vi "Create Path URL.vi"(6 "Weight":i32=5, 7 "Path Collor":u32(colorbox)=16715776, 8 "Long Point 2":string, 9 "Lat Point 2":string, 10 "Long Point 1":string, 11 "Lat Point 1":string) -> (3 "String 4":string)   [LabVIEW 2012]
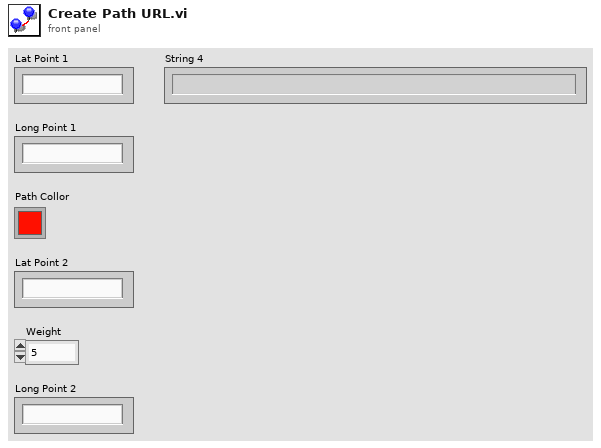
[diagram p1: front panel]
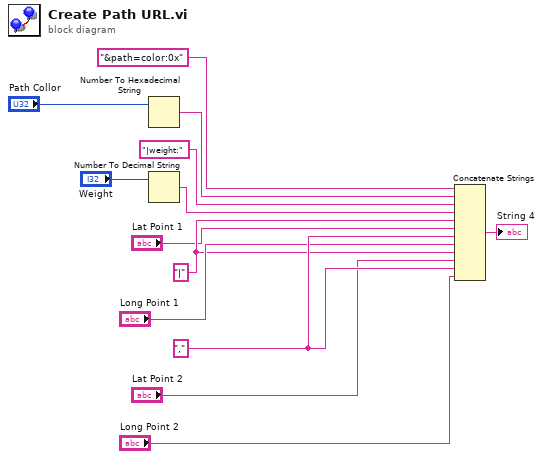
[diagram p0: block diagram]
diagram:
  w13 = "," ("string")
  w11 = "|"
  n1 = Number To Hexadecimal String(2:"Path Collor") -> (0:w3:string)  [unwired: 1 in]
  n2 = Number To Decimal String(number="Weight") -> (decimal integer string=w6:string)  [unwired: 1 in]
  n3 = Concatenate Strings("&path=color:0x" ("string"), w3, "|weight:", w6, w11, "Lat Point 1", w13, "Long Point 1", w11, "Lat Point 2", w13, "Long Point 2") -> (→"String 4":string)
